vi "GarbleString.vi"(10 "String In":string) -> (2 "String Out":string)   [LabVIEW 2015, in "SystemLink File configuration.lvclass"]
doc: "THIS VI IS TO PREVENT SAVING PLAINTEXT PASSWORDS BUT IS NOT SECURE IN ANY WAY. THIS IS A PLACEHOLDER THAT SHOULD BE REPLACED"
uses:
  SystemLink File configuration.lvclass
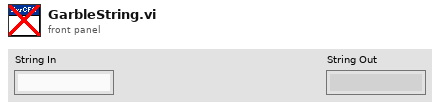
[diagram p1: front panel]
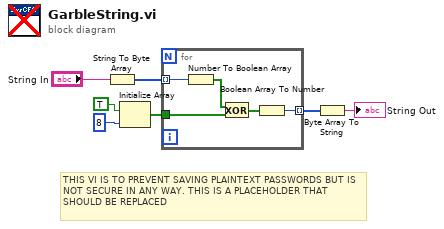
[diagram p0: block diagram]
diagram:
  # "THIS VI IS TO PREVENT SAVING PLAINTEXT PASSWORDS BUT IS NOT SECURE IN ANY WAY. THIS IS A PLACEHOLDER THAT SHOULD BE REPLACED"
  n1 = String To Byte Array(string="String In") -> (unsigned byte array=w7:u8[])
  n2 = Initialize Array(TRUE, 8 ("dimension size")) -> (w4:bool[])
  n3 = for {
    tunnel: w7 -> [w12] mode=indexing
    tunnel: w4 -> [w10]
    tunnel: [w8] -> w3 mode=indexing
    n4 = Number To Boolean Array(number=w12) -> (Boolean array=w11:bool[])
    n5 = Exclusive Or(1:w10, 2:w11) -> (0:w9:bool[])
    n6 = Boolean Array To Number(Boolean array=w9) -> (number=w8:u8)
  }
  n7 = Byte Array To String(unsigned byte array=w3) -> (string=→"String Out":string)
